vi "Measurement UI.vi"() -> ()   [LabVIEW 2025, in "Ni-Scope-Multirecords UI.lvlib"]
uses:
  Ni-Scope-Multirecords UI.lvlib
panel:
  out "Waveform Graph":T1(graph)
  in  "Stream To File Path":path caption="Stream To File Path (Optional)"
  in  "Get Configuration in File":bool
  in  "Record Length":dbl=100.0 format="%#_6p%"
  in  "Length Unit":string(combo)="Percentage"
  in  "Trigger Position":dbl format="%#_6ps"
  in  "Delay Mode":string(combo)="On"
  out "Actual Record Duration":dbl format="%#_6ps"
  out "Actual Sample Rate":dbl format="%#_6pHz"
  out "Actual Record Length":dbl format="%#_6p Samples"
  in  "Configuration File Path":path
  in  "Timeout (s)":dbl=5.0 format="%#_6p"
  in  "Number Of Records":i32=2
  in  "Resource Name(s)":string[](array[combo])
  out "Wfm":dbl[][](array[numeric])
  out "xIncrement":dbl[](array[numeric])
  out "RelativeInitialX":dbl[](array[numeric])
  # "Configuration Changes"
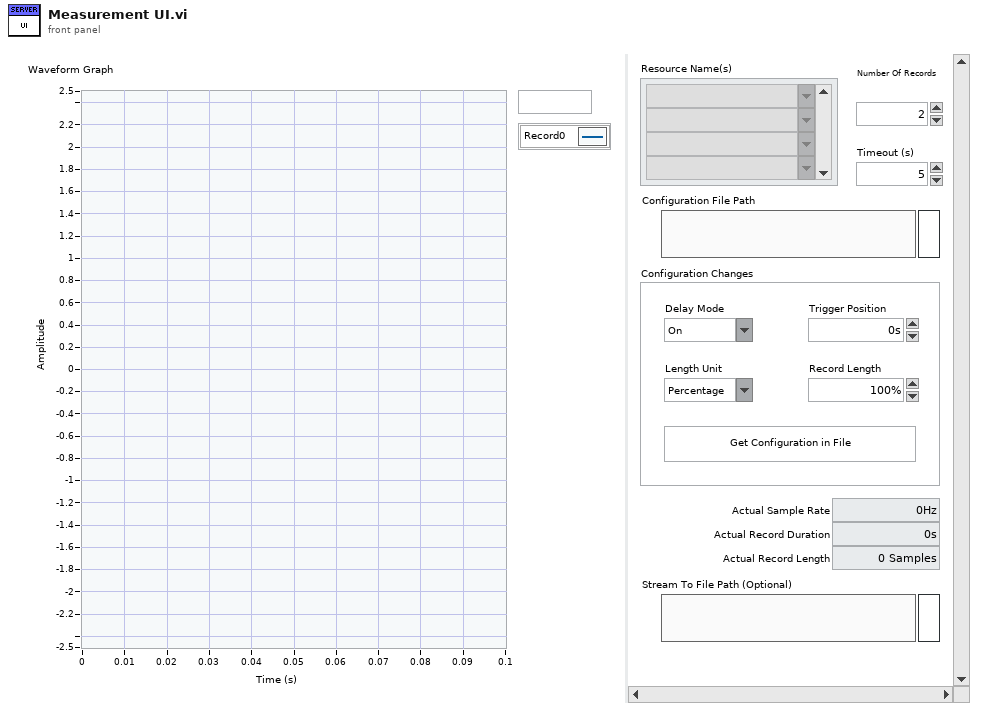
[diagram p1: front panel]
types:
  T1 = cluster{"relativeInitialX":dbl, "xIncrement":dbl, "wfm":dbl[]}[]
  T2 = cluster{"Numeric":dbl, "Numeric":dbl, "Value":dbl[]}
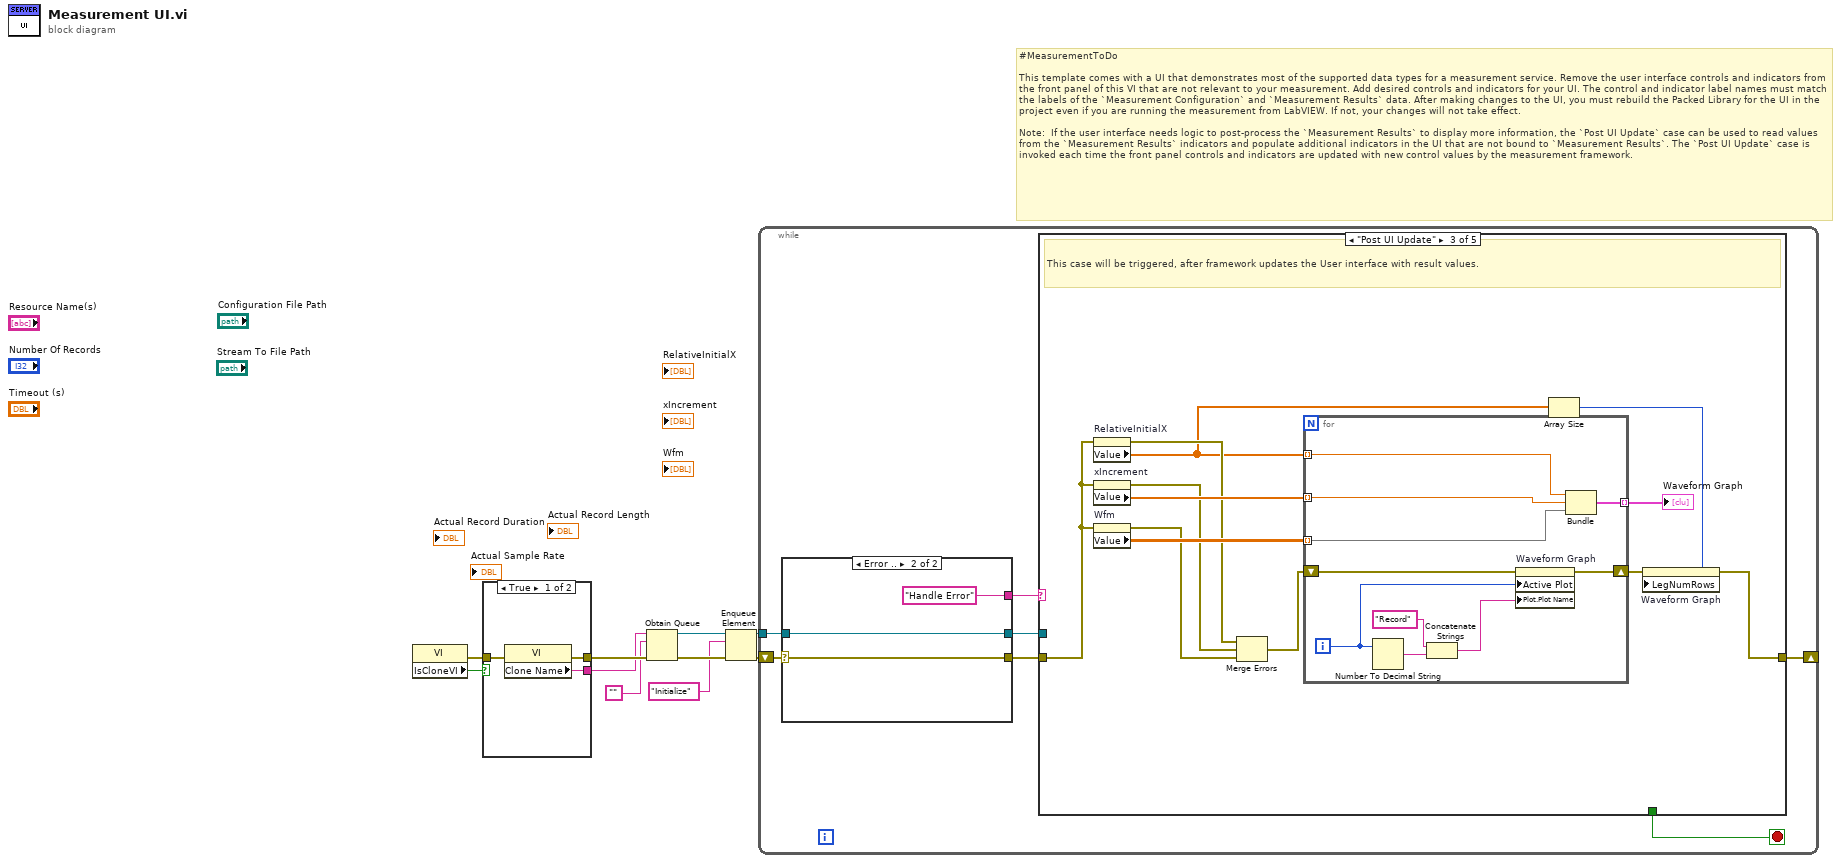
[diagram p0: block diagram]
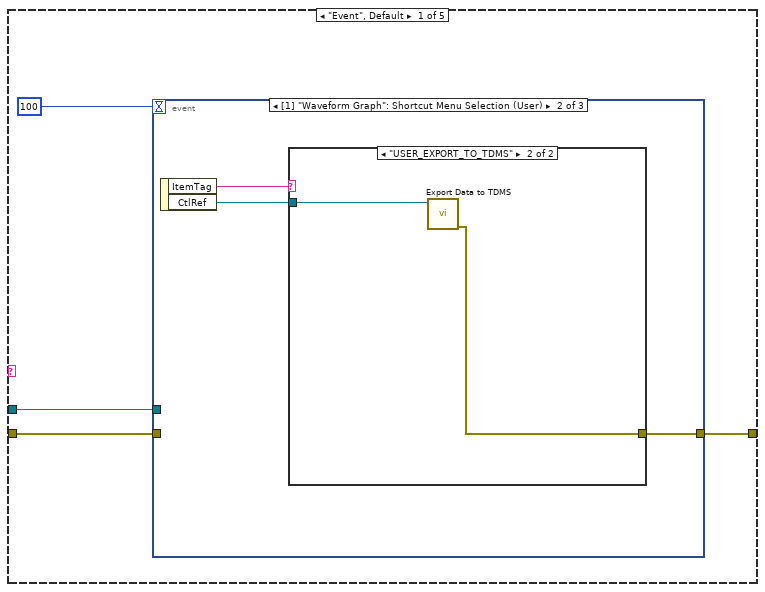
[diagram p2: hidden frame]
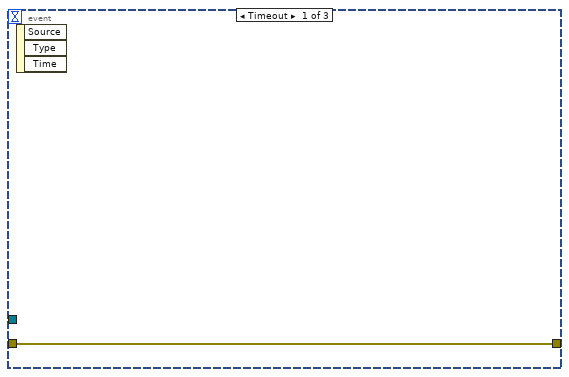
[diagram p3: hidden frame]
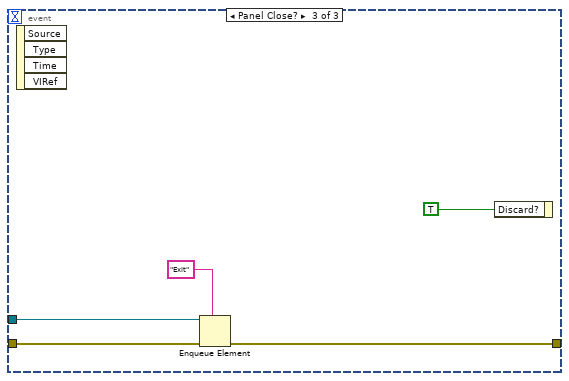
[diagram p5: hidden frame]
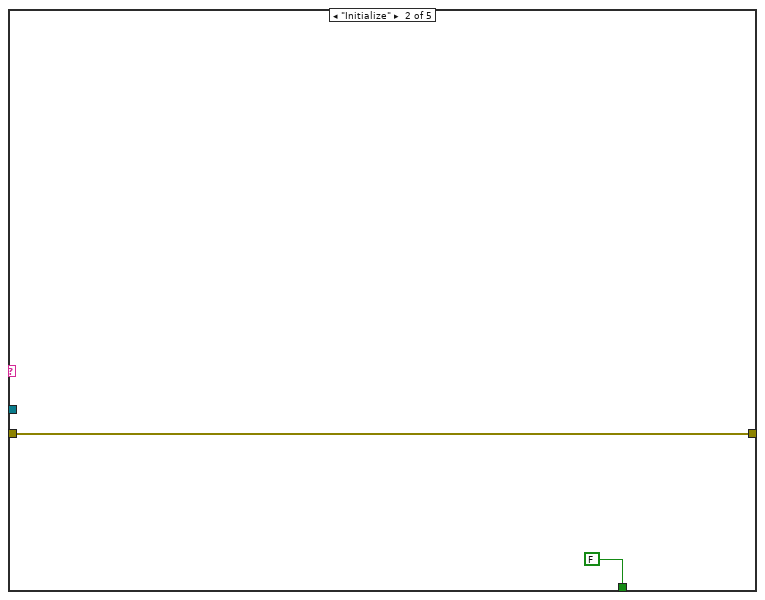
[diagram p6: hidden frame]
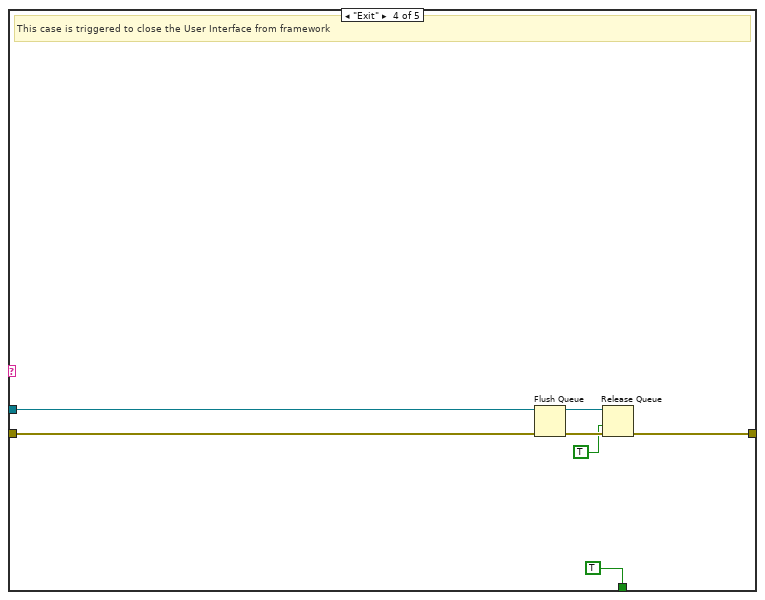
[diagram p7: hidden frame]
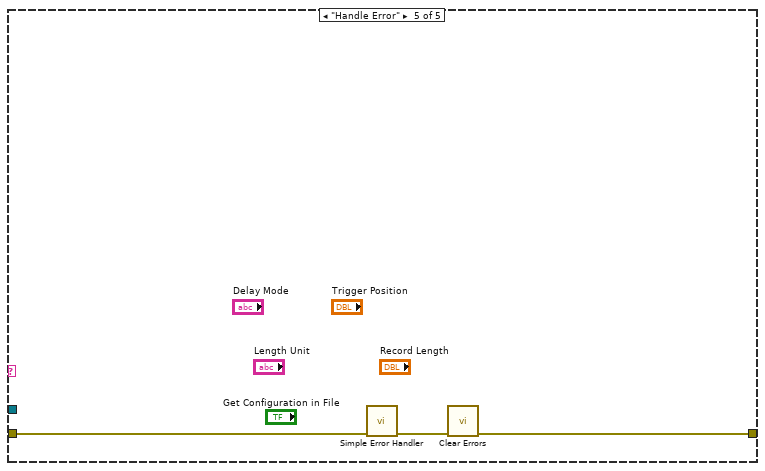
[diagram p8: hidden frame]
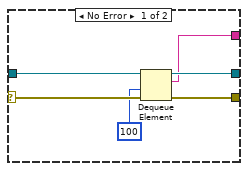
[diagram p9: hidden frame]
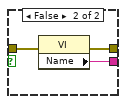
[diagram p10: hidden frame]
diagram:
  # "#MeasurementToDo  \n\nThis template comes with a UI that demonstrates most of the supported data types for a measurement service. Remove the user interface controls and indicators from the front panel of this VI that are not relevant to your measurement. Add desired controls and indicators for your UI. The control and indicator label names must match the labels of the `Measurement Configuration` and `Measurement Results` data. After making changes to the UI, you must rebuild the Packed Library for the UI in the project even if you are running the measurement from LabVIEW. If not, your changes will not take effect.\n\nNote:  If the user interface needs logic to post-process the `Measurement Results` to display more information, the `Post UI Update` case can be used to read values from the `Measurement Results` indicators and populate additional indicators in the UI that are not bound to `Measurement Results`. The `Post UI Update` case is invoked each time the front panel controls and indicators are updated with new control values by the measurement framework."
  n1 = property class="VI"() -> (error out=w1:errorcluster, "IsCloneVI"=w2:bool)  [unwired: 2 in, 1 out]
  n2 = case shown="True" w2 {
    tunnel: [w13 w16] -> w10
    tunnel: [w12 w15] -> w9
    tunnel: w1 -> [w11 w14]
    frame True {
      n3 = property class="VI"(error in=w11) -> (error out=w13:errorcluster, "Clone Name"=w12:string)  [unwired: 1 in, 1 out]
    }
    frame False {
      n4 = property class="VI"(error in=w14) -> (error out=w16:errorcluster, "Name"=w15:string)  [unwired: 1 in, 1 out]
    }
  }
  n5 = Obtain Queue(name (unnamed)=w9, element data type="", error in (no error)=w10) -> (queue out=w6:refnum<queue>, error out=w8:errorcluster)  [unwired: 2 in, 1 out]
  n6 = Enqueue Element(queue=w6, element="Initialize", error in (no error)=w8) -> (queue out=w5:refnum<queue>, error out=w7:errorcluster)  [unwired: 1 in, 1 out]
  n7 = while {
    shift-right: [w18] -> _
    shift-left: w7 -> [w23]
    tunnel: w5 -> [w21]
    stop <- w17 stop-if-true
    n8 = case shown="Error .." w23 {
      selector: w23 -> [w78 w81]
      tunnel: [w77 w81] -> w22
      tunnel: w21 -> [w76 w80]
      tunnel: [w75 w80] -> w20
      tunnel: [w74 "Handle Error"] -> w19
      frame No Error {
        n9 = Dequeue Element(queue=w76, timeout in ms (-1)=100, error in (no error)=w78) -> (queue out=w75:refnum<queue>, element=w74:string, error out=w77:errorcluster)  [unwired: 1 out]
      }
      frame Error {
      }
    }
    n10 = case shown="\"Post UI Update\"" w19 {
      tunnel: w22 -> [w26 w40 w49 w69 w72]
      tunnel: w20 -> [w24 _ _ w67 _]
      tunnel: [w27 w40 w42 w64 w70] -> w18
      tunnel: [_ FALSE _ TRUE _] -> w17
      frame "Event", Default {
        n11 = event shown="[1] \"Waveform Graph\": Shortcut Menu Selection (User)" {
          selector: _ -> [_ _ _]
          dyn-events: _ -> [_ _ _]
          timeout: 100 -> [_ _ _]
          tunnel: [w28 w29 w36] -> w27
          tunnel: w26 -> [w28 _ w37]
          tunnel: w24 -> [_ _ w35]
          event Timeout {
            n12 = event-data() -> ()  [unwired: 1 in, 3 out]
          }
          event "Waveform Graph": Shortcut Menu Selection (User) {
            n13 = event-data() -> ("ItemTag"=w31:string, "CtlRef"=w30:refnum<vi>)  [unwired: 1 in]
            n14 = case shown="\"USER_EXPORT_TO_TDMS\"" w31 {
              tunnel: w30 -> [_ w33]
              tunnel: [_ w32] -> w29
              frame "False", Default {
              }
              frame "USER_EXPORT_TO_TDMS" {
                n15 = call "Export Data to TDMS.vi"("WaveformGraph in"=w33) -> ("error out"=w32:errorcluster)  [unwired: 10 in]
              }
            }
          }
          event Panel Close? {
            n16 = event-data() -> ()  [unwired: 1 in, 4 out]
            n17 = Enqueue Element(queue=w35, element="Exit", error in (no error)=w37) -> (error out=w36:errorcluster)  [unwired: 1 in, 2 out]
            n18 = event-data("Discard?"=TRUE) -> ()  [unwired: 1 in, 1 out]
          }
        }
      }
      frame "Initialize" {
      }
      frame "Post UI Update" {
        # "This case will be triggered, after framework updates the User interface with result values."
        n19 = property on="RelativeInitialX" class="Arr (strict)"(error in=w49) -> (error out=w46:errorcluster, "Value"=w45:dbl[])  [unwired: 1 in, 1 out]
        n20 = property on="xIncrement" class="Arr (strict)"(error in=w49) -> (error out=w47:errorcluster, "Value"=w52:dbl[])  [unwired: 1 in, 1 out]
        n21 = property on="Wfm" class="Arr (strict)"(error in=w49) -> (error out=w48:errorcluster, "Value"=w51:dbl[][])  [unwired: 1 in, 1 out]
        n22 = Merge Errors(w46, w47, w48) -> (w44:errorcluster)
        n23 = for {
          tunnel: w45 -> [w62] mode=indexing
          tunnel: w52 -> [w61] mode=indexing
          tunnel: w51 -> [w60] mode=indexing
          tunnel: [w59] -> w50 mode=indexing
          shift-right: [w53] -> w43
          shift-left: w44 -> [w54]
          i -> [w55]
          n24 = Number To Decimal String(number=w55) -> (decimal integer string=w57:string)  [unwired: 1 in]
          n25 = Concatenate Strings("Record", w57) -> (w56:string)
          n26 = property on="Waveform Graph" class="WFGraph (strict)"(error in=w54, "Active Plot"=w55, "Plot.Plot Name"=w56) -> (error out=w53:errorcluster)  [unwired: 1 in, 1 out]
          n27 = Bundle("Numeric"=w62, "Numeric"=w61, "Value"=w60) -> (w59:T2)  [unwired: 1 in]
        }
        "Waveform Graph" <- w50
        n28 = Array Size(array=w45) -> (size(s)=w41:i32)
        n29 = property on="Waveform Graph" class="WFGraph (strict)"(error in=w43, "LegNumRows"=w41) -> (error out=w42:errorcluster)  [unwired: 1 in, 1 out]
      }
      frame "Exit" {
        # "This case is triggered to close the User Interface from framework"
        n30 = Flush Queue(queue=w67, error in (no error)=w69) -> (queue out=w66:refnum<queue>, error out=w65:errorcluster)  [unwired: 1 out]
        n31 = Release Queue(queue=w66, force destroy? (F)=TRUE, error in (no error)=w65) -> (error out=w64:errorcluster)  [unwired: 2 out]
      }
      frame "Handle Error" {
        n32 = call <vilib>:"Simple Error Handler.vi"("error in (no error)"=w72) -> ("error out"=w71:errorcluster)  [unwired: 4 in, 4 out]
        n33 = call <vilib>:"Clear Errors.vi"("error in (no error)"=w71) -> ("error out"=w70:errorcluster)  [unwired: 5 in, 1 out]
      }
    }
  }
